vi "Check-position.vi"(8 "error in (no error)":errorcluster, 10 "Position in":dbl caption="Position [unit]", 11 "Motor-Serial in":refnum<class "Motor-Serial.lvclass">) -> (0 "error out":errorcluster, 1 "In range?":bool, 2 "Position out":dbl caption="Position out [unit]", 3 "Motor-Serial out":refnum<class "Motor-Serial.lvclass">)   [LabVIEW 2013, in "PowderDeposition.lvlib" / "Motor-Serial.lvclass"]
uses:
  Motor-Serial.lvclass
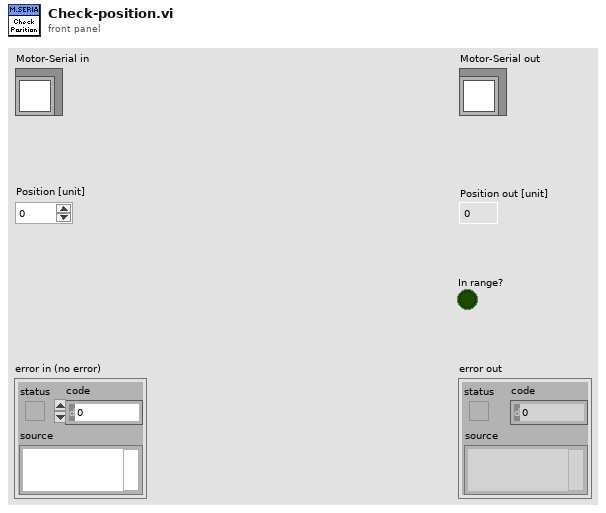
[diagram p1: front panel]
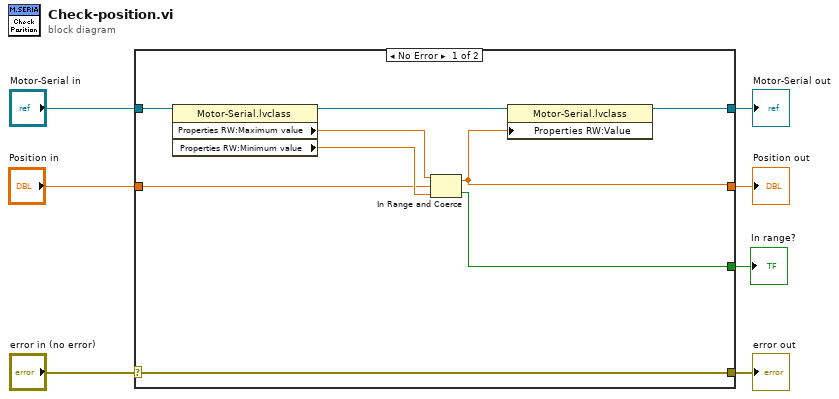
[diagram p0: block diagram]
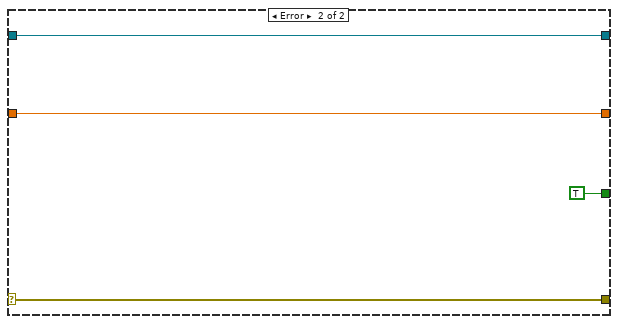
[diagram p2: hidden frame]
diagram:
  n1 = case shown="No Error" "error in (no error)" {
    selector: "error in (no error)" -> [w15 w20]
    tunnel: [w15 w20] -> w6
    tunnel: [w9 w19] -> w4
    tunnel: "Motor-Serial in" -> [w16 w19]
    tunnel: "Position in" -> [w10 w18]
    tunnel: [w8 w18] -> w2
    tunnel: [w11 TRUE] -> w1
    frame No Error {
      n2 = property class="Motor-Serial.lvclass"(reference=w16) -> (reference out=w14:refnum<class "Motor-Serial.lvclass">, "Properties RW:Maximum value"=w12:dbl, "Properties RW:Minimum value"=w13:dbl)  [unwired: 1 in, 1 out]
      n3 = In Range and Coerce(upper limit=w12, x=w10, lower limit=w13) -> (coerced(x)=w8:dbl, In Range?=w11:bool)
      n4 = property class="Motor-Serial.lvclass"(reference=w14, "Properties RW:Value"=w8) -> (reference out=w9:refnum<class "Motor-Serial.lvclass">)  [unwired: 1 in, 1 out]
    }
    frame Error {
    }
  }
  "error out" <- w6
  "Motor-Serial out" <- w4
  "Position out" <- w2
  "In range?" <- w1
